vi "Example - Simple.vi"() -> ()   [LabVIEW 2017]
uses:
  DI_class/DI.lvclass
panel:
  out "DI Channel Status":bool
  in  "DI Channel Number (Zero Based)":i32
  out "All DI Status":bool[](array[boolean])
  in  "Quit Program":bool
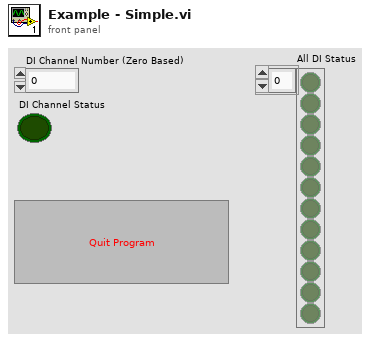
[diagram p1: front panel]
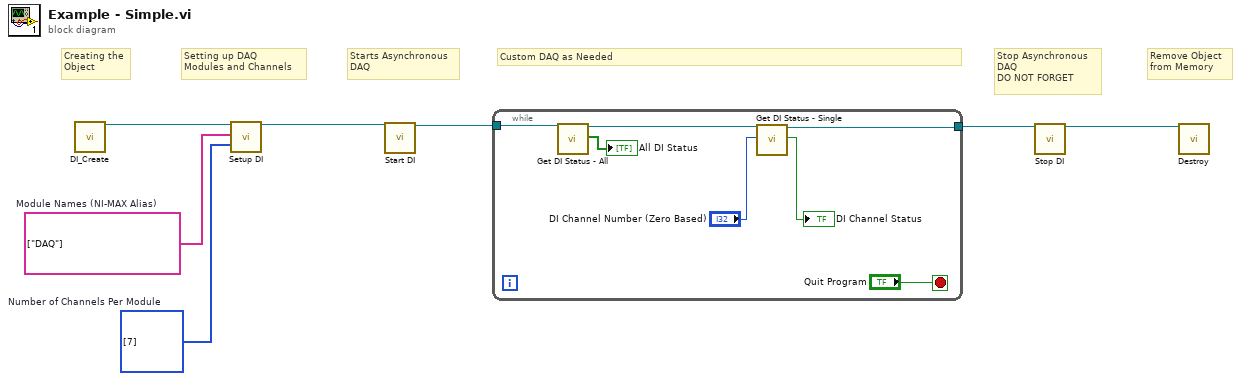
[diagram p0: block diagram]
diagram:
  w2 = u32[] [7]  # Number of Channels Per Module
  w1 = string[] ["DAQ"]  # Module Names (NI-MAX Alias)
  # "Creating the\nObject"
  # "Setting up DAQ\nModules and Channels"
  # "Custom DAQ as Needed"
  # "Remove Object\nfrom Memory"
  # "Stop Asynchronous\nDAQ\nDO NOT FORGET"
  # "Starts Asynchronous\nDAQ"
  n1 = call "DI_Create.vi"() -> ("reference out"=w7:refnum<class "DI.lvclass">)  [unwired: 18 in, 1 out]
  n2 = call-dynamic "Setup DI.vi"("reference in"=w7, "Module Names (NI-MAX Alias)"=w1, "Number of Channels Per Module"=w2) -> ("reference out"=w6:refnum<class "DI.lvclass">)  [unwired: 15 in, 1 out]
  n3 = call-dynamic "Start DI.vi"("reference in"=w6) -> ("reference out"=w5:refnum<class "DI.lvclass">)  [unwired: 17 in, 1 out]
  n4 = while {
    tunnel: w5 -> [w13]
    tunnel: [w11] -> w4
    stop <- "Quit Program" stop-if-true
    n5 = call-dynamic "Get DI Status - All.vi"("reference in"=w13) -> ("reference out"=w12:refnum<class "DI.lvclass">, "All DI Status"=→"All DI Status":bool[])  [unwired: 16 in, 1 out]
    n6 = call-dynamic "Get DI Status - Single.vi"("reference in"=w12, "DI Channel Number (Zero Based)"="DI Channel Number (Zero Based)") -> ("reference out"=w11:refnum<class "DI.lvclass">, "DI Channel Status"=→"DI Channel Status":bool)  [unwired: 14 in, 2 out]
  }
  n7 = call-dynamic "Stop DI.vi"("reference in"=w4) -> ("reference out"=w3:refnum<class "DI.lvclass">)  [unwired: 17 in, 1 out]
  n8 = call-dynamic "Destroy.vi"("reference in"=w3) -> ()  [unwired: 17 in, 2 out]
